vi "Error - Fire Event.vi"(8 "error in (no error)":errorcluster, 9 "Error Data":variant, 10 "Error Level":T1, 11 "View Model":T2) -> (0 "error out":errorcluster)   [LabVIEW 2017]
doc: "Generate Error Message user event with additional data."
uses:
  View Model/Controls/View Model.ctl
  View Model/Controls/Shared Model.ctl
  Controls/Error Model.ctl
  Controls/Error Message.ctl
  Controls/Error Level.ctl
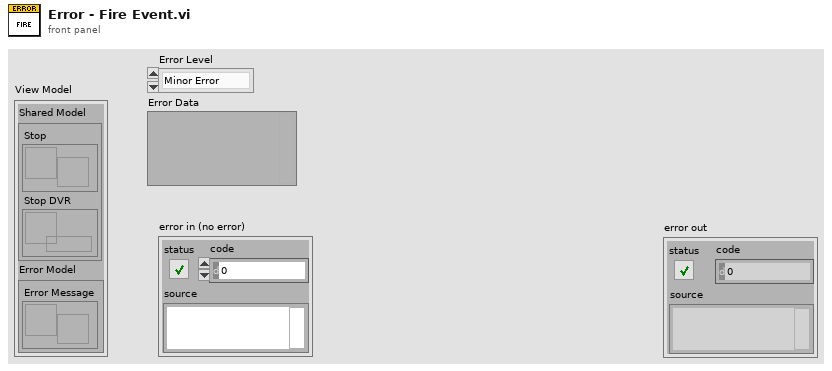
[diagram p1: front panel]
types:
  T1 = typedef "Error Level.ctl" = enum16{"Minor Error", "Wash Cycle Error", "System Error"}
  T2 = typedef "View Model.ctl" = cluster{"Shared Model":T3, "Error Model":T4}
  T3 = typedef "Shared Model.ctl" = cluster{"Stop":refnum<user-event>, "Stop DVR":refnum<data-value>}
  T4 = typedef "Error Model.ctl" = cluster{"Error Message":refnum<user-event>}
  T5 = typedef "Error Message.ctl" = cluster{"Error Level":T1, "Error Data":variant}
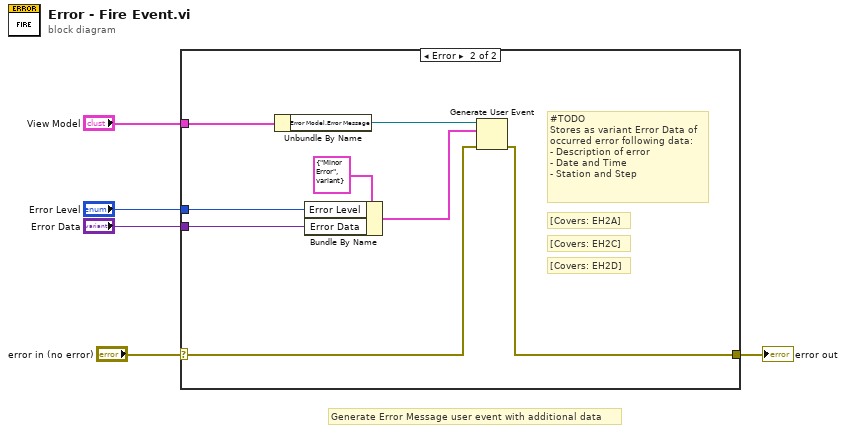
[diagram p0: block diagram]
diagram:
  # "Generate Error Message user event with additional data"
  n1 = case shown="Error" "error in (no error)" {
    selector: "error in (no error)" -> [w6 w12]
    tunnel: [w6 w7] -> w4
    tunnel: "View Model" -> [_ w14]
    tunnel: "Error Data" -> [_ w9]
    tunnel: "Error Level" -> [_ w8]
    frame No Error {
    }
    frame Error {
      # "[Covers: EH2D]"
      # "[Covers: EH2C]"
      # "[Covers: EH2A]"
      # "#TODO\nStores as variant Error Data of\noccurred error following data:\n- Description of error\n- Date and Time\n- Station and Step"
      n2 = Unbundle By Name(w14) -> ("Error Model.Error Message"=w13:refnum<user-event>)
      n3 = Bundle By Name(cluster=T5 {"Error Level"=enum."Minor Error", "Error Data"=variant} ("Error Message"), "Error Level"=w8, "Error Data"=w9) -> (w10:T5)
      n4 = Generate User Event(user event=w13, event data cluster=w10, error in=w12) -> (error out=w7:errorcluster)  [unwired: 1 in, 1 out]
    }
  }
  "error out" <- w4
